vi "Update All.vi"(0 "reference in":refnum<class "SSR.lvclass">, 5 "error in (no error)":errorcluster) -> (14 "reference out":refnum<class "SSR.lvclass">, 19 "error out":errorcluster)   [LabVIEW 2017, in "SSR.lvclass"]
uses:
  SSR.lvclass
  <vilib>/DAQmx/write.llb/DAQmx Write (Digital 1D Bool NChan 1Samp 1Line).vi
  <vilib>/DAQmx/miscellaneous.llb/DAQmx Fill In Error Info.vi
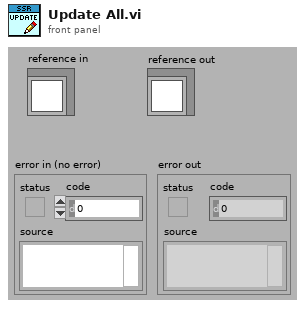
[diagram p1: front panel]
types:
  T1 = typedef "SSR.lvclass/ObjectAttributes.ctl" = cluster{"SSR Task":refnum<k21>, "SSR On/Off Status":bool, "Number of SSR Modules":u32, "Number of Total SSR Channels":u32, "SSR Module Names (NI-Max Name)":string[], "Number of Channels Per SSR Module":i32[], "SSR Status":bool[], "SSR Status to Set":bool[], "SSR VI Reference":refnum<vi>}
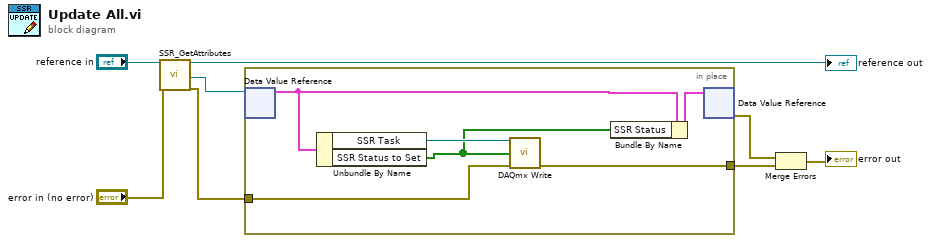
[diagram p0: block diagram]
diagram:
  n1 = call "SSR_GetAttributes.vi"("reference in"="reference in", "error in (no error)"="error in (no error)") -> ("reference out"=→"reference out":refnum<class "SSR.lvclass">, "DataRef"=w3:refnum<data-value>, "error out"=w2:errorcluster)  [unwired: 14 in, 1 out]
  n2 = in-place {
    in-place-border: w2 -> [w10]
    in-place-border: [w9] -> w1
    n3 = in-place-dvr #1(w3) -> (w11:T1)  [unwired: 1 out]
    n4 = Unbundle By Name(w11) -> ("SSR Task"=w13:refnum<k21>, "SSR Status to Set"=w12:bool[])
    n5 = call-poly <vilib>:"DAQmx Write.vi"("task/channels in"=w13, "data"=w12, "error in"=w10) -> ("error out"=w9:errorcluster)  [unwired: 10 in, 2 out]
    n6 = Bundle By Name(cluster=w11, "SSR Status"=w12) -> (w14:T1)
    n7 = in-place-dvr #1(w14) -> (w4:errorcluster)  [unwired: 1 out]
  }
  n8 = Merge Errors(w4, w1) -> (→"error out":errorcluster)
